vi "Handle Exit.vi"(8 "error in (no error)":errorcluster, 9 "Stop Argument":T1, 10 "Module Admin in":refnum<class "Delacor_lib_QMH_Cloneable Module Admin.lvclass">, 11 "VI reference":refnum<vi>) -> (0 "error out":errorcluster, 3 "Wait for Stop?":bool)   [LabVIEW 2015, in "ModbusOverMOXA.lvlib"]
doc: "This VI handles the Exit Message for a DQMH Cloneable module. \n\nThis VI determines if the message was received via the Stop Request or not. If the Exit message was received via the Request Event to Stop the module then there is no need to send the Stop Request again. If it was not, then the Stop Request needs to be fired so the Event Handling Loop can stop.\n\nThis VI also hides the Main.vi Front Panel, this is to ensure that the module stays in memory until the very last step in the Main.vi which is to close the front panel.\n\n_____\nBased on Delacor QMH Project Template 3.1.0.34."
uses:
  ModbusOverMOXA.lvlib
  Stop Argument--cluster.ctl
  <vilib>/Delacor/Delacor QMH/Libraries/Cloneable Module Admin_class/Delacor_lib_QMH_Cloneable Module Admin.lvclass
  <vilib>/Delacor/Delacor QMH/Libraries/Cloneable Module Admin_class/Delacor_lib_QMH_Cloneable Module Admin.lvclass/Delacor_lib_QMH_Cloneable Module Admin.ctl
  <vilib>/Delacor/Delacor QMH/Libraries/Module Admin_class/Delacor_lib_QMH_Module Admin.lvclass/Delacor_lib_QMH_Module Admin.ctl
  <vilib>/Delacor/Delacor QMH/Libraries/Cloneable Module Admin_class/Delacor_lib_QMH_Get Module ID.vi
  <vilib>/Delacor/Delacor QMH/Libraries/Module Admin_class/Delacor_lib_QMH_Get External Launch.vi
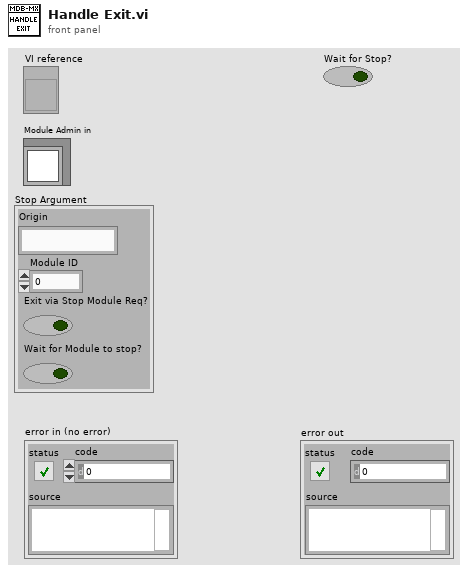
[diagram p1: front panel]
types:
  T1 = typedef "ModbusOverMOXA.lvlib/Stop Argument--cluster.ctl" = cluster{"Origin":string, "Module ID":i32, "Exit via Stop Module Req?":bool, "Wait for Module to stop?":bool}
  T2 = enum32{"Invalid", "Standard", "Closed", "Hidden", "Minimized", "Maximized"}
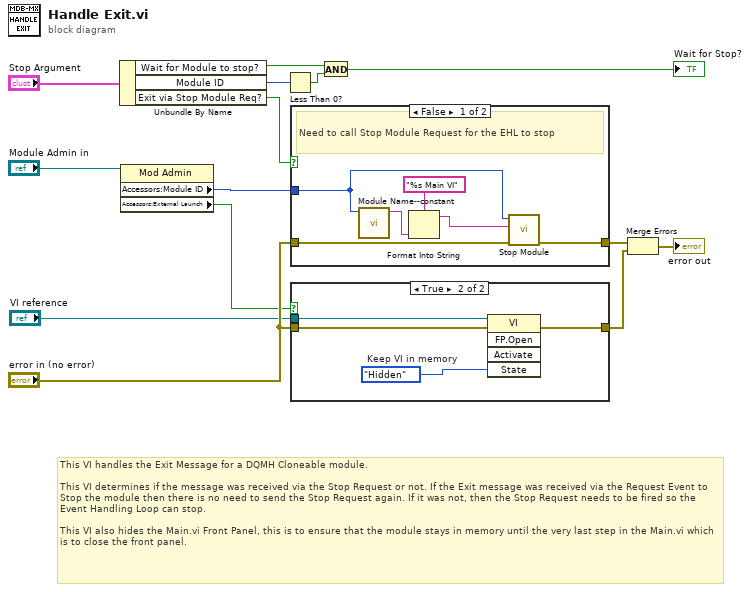
[diagram p0: block diagram]
diagram:
  # "This VI handles the Exit Message for a DQMH Cloneable module. \n\nThis VI determines if the message was received via the Stop Request or not. If the Exit message was received via the Request Event to Stop the module then there is no need to send the Stop Request again. If it was not, then the Stop Request needs to be fired so the Event Handling Loop can stop.\n\nThis VI also hides the Main.vi Front Panel, this is to ensure that the module stays in memory until the very last step in the Main.vi which is to close the front panel."
  n1 = Unbundle By Name("Stop Argument") -> ("Wait for Module to stop?"=w12:bool, "Module ID"=w10:i32, "Exit via Stop Module Req?"=w9:bool)
  n2 = property class="Mod Admin"(reference="Module Admin in") -> ("Accessors:Module ID"=w6:i32, "Accessors:External Launch"=w4:bool)  [unwired: 1 in, 2 out]
  n3 = Less Than 0?(x=w10) -> (x < 0?=w11:bool)
  n4 = case "Exit came from Stop Module Request?" shown="False" w9 {
    tunnel: [w18 w21] -> w7
    tunnel: w6 -> [w16 _]
    tunnel: "error in (no error)" -> [w15 w21]
    frame False {
      # "Need to call Stop Module Request for the EHL to stop"
      n5 = call "Module Name--constant.vi"("Module ID"=w16) -> ("Module Name"=w17:string)  [unwired: 10 in]
      n6 = Format Into String(format string="%s Main VI", w17) -> (resulting string=w19:string)  [unwired: 2 in, 1 out]
      n7 = call "Stop Module.vi"("error in (no error)"=w15, "Origin"=w19, "Module ID"=w16) -> ("error out"=w18:errorcluster)  [unwired: 8 in]
    }
    frame True {
      # "no need to call Stop Module Request again."
    }
  }
  n8 = case shown="True" w4 {
    tunnel: "VI reference" -> [_ w26]
    tunnel: "error in (no error)" -> [w22 w25]
    tunnel: [w22 w24] -> w1
    frame False {
    }
    frame True {
      w23 = T2."Hidden"  # Keep VI in memory
      n9 = invoke class="VI" method="FP.Open"(reference=w26, error in=w25, "State"=w23) -> (error out=w24:errorcluster)  [unwired: 2 in, 4 out]
    }
  }
  n10 = And(x=w12, y=w11) -> (x .and. y?=→"Wait for Stop?":bool)
  n11 = Merge Errors(w7, w1) -> (→"error out":errorcluster)
